vi "test1-HexStr conversion.vi"(8 "error in (no error)":errorcluster, 11 "TestCase in":refnum<class "testcase-CSMArgument.lvclass">) -> (0 "error out":errorcluster, 3 "TestCase out":refnum<class "testcase-CSMArgument.lvclass">)   [LabVIEW 2017, in "testcase-CSMArgument.lvclass"]
uses:
  testcase-CSMArgument.lvclass
  <vilib>/addons/_JKI Toolkits/VI Tester/TestCase.llb/TestCase.lvclass
  src/user.lib/_NEVSTOP/Communicable State Machine(CSM)/Communicable State Machine.lvlib
  src/user.lib/_NEVSTOP/Communicable State Machine(CSM)/_Shared/CSM Shared.lvlib
  CSM/CSM-Testcase.lvlib
  C:/Program Files (x86)/National Instruments/LabVIEW 2017/vi.lib/addons/_JKI Toolkits/VI Tester/TestCase.llb/TestCase.lvclass
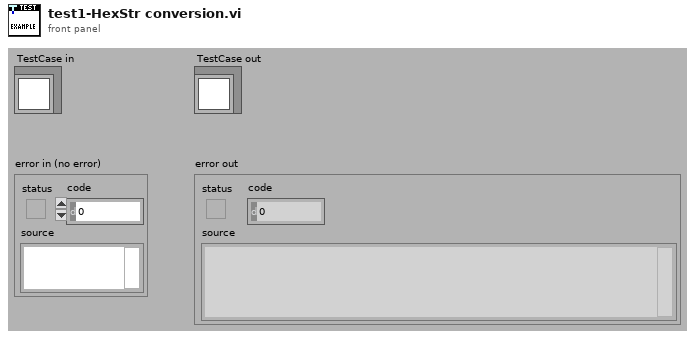
[diagram p1: front panel]
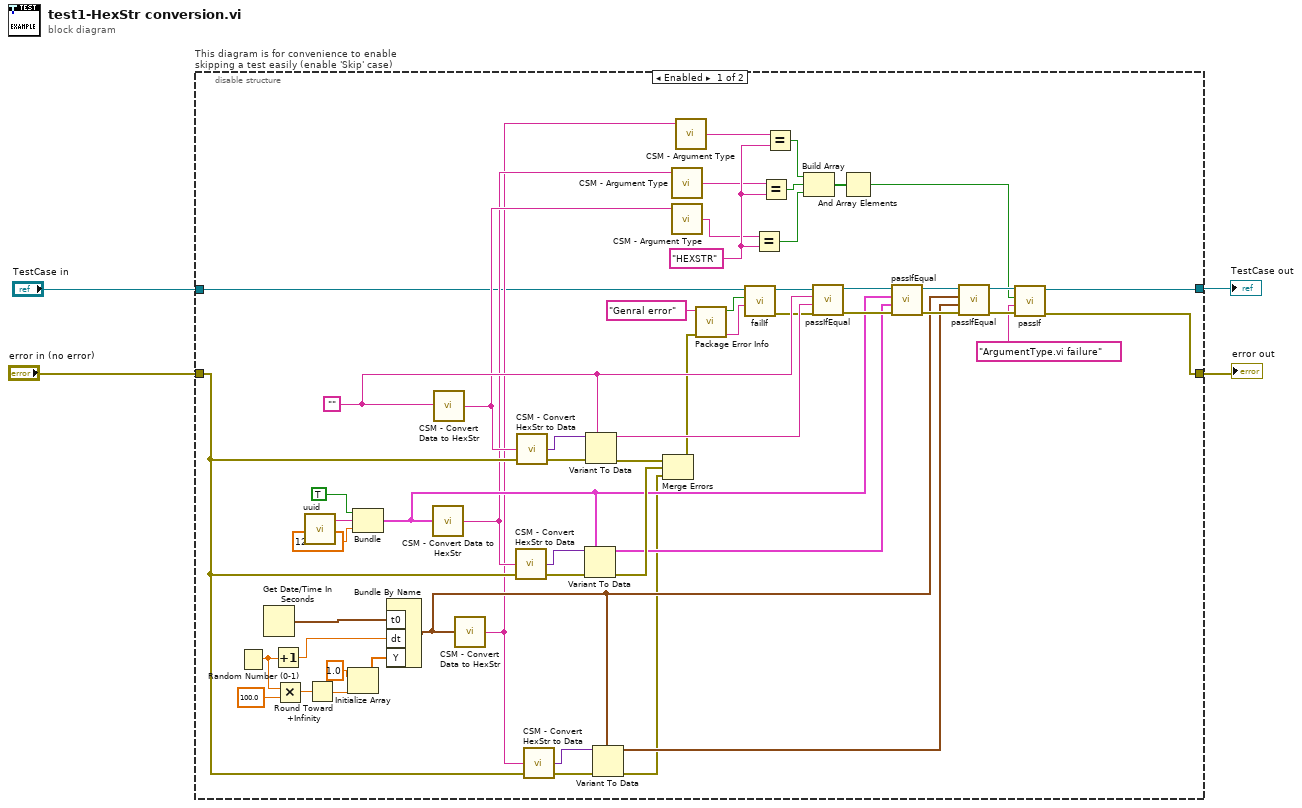
[diagram p0: block diagram]
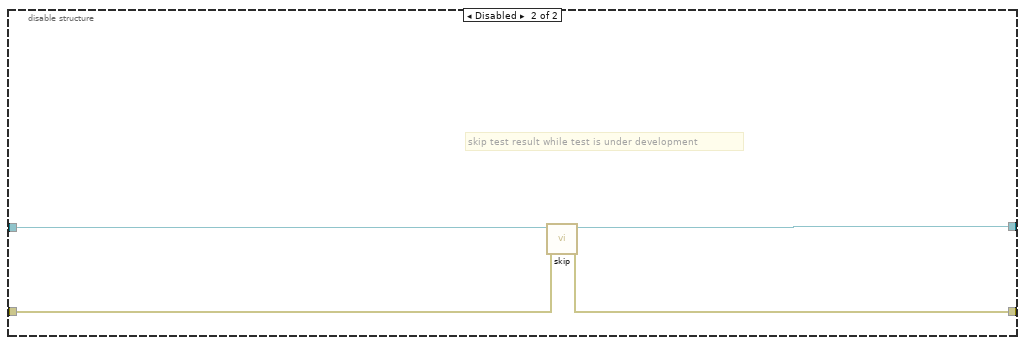
[diagram p2: hidden frame]
diagram:
  n1 = disable-structure "This diagram is for convenience to enable skipping a test easily (enable 'Skip' case)" shown="Enabled" {
    disable-tunnel: "TestCase in" -> [w11 w63]
    disable-tunnel: [w19 w61] -> w1
    disable-tunnel: [w17 w62] -> w3
    disable-tunnel: "error in (no error)" -> [w42 w60]
    frame Enabled {
      w25 = "HEXSTR"
      w53 = ""
      n2 = Random Number (0-1)() -> (number: 0 to 1=w38:dbl)
      n3 = Get Date/Time In Seconds() -> (seconds since 1Jan1904=w41:timestamp)
      n4 = Increment(x=w38) -> (x+1=w40:dbl)
      n5 = Multiply(x=w38, y=100.0) -> (x*y=w36:dbl)
      n6 = call "uuid.vi"() -> ("UUID"=w58:string)  [unwired: 11 in]
      n7 = Round Toward +Infinity(x=w36) -> (ceil(x): smallest int >= x=w35:dbl)
      n8 = Initialize Array(1.0 ("element"), w35) -> (w34:dbl[])
      n9 = Bundle(TRUE, "UUID"=w58, 123.456) -> (w46:cluster{bool, "UUID":string, dbl})  [unwired: 1 in]
      n10 = Bundle By Name("t0"=w41, "dt"=w40, "Y"=w34) -> (w31:waveform(dbl))  [unwired: 1 in]
      n11 = call "CSM - Convert Data to HexStr.vi"("Variant"=w46) -> ("HEX String (0-9,A-F)"=w27:string)  [unwired: 8 in]
      n12 = call "CSM - Convert Data to HexStr.vi"("Variant"=w53) -> ("HEX String (0-9,A-F)"=w28:string)  [unwired: 8 in]
      n13 = call "CSM - Convert Data to HexStr.vi"("Variant"=w31) -> ("HEX String (0-9,A-F)"=w26:string)  [unwired: 8 in]
      n14 = call "CSM - Convert HexStr to Data.vi"("HEX String"=w27, "error in (no error)"=w42) -> ("Variant"=w49:variant, "error out"=w51:errorcluster)  [unwired: 6 in]
      n15 = call "CSM - Convert HexStr to Data.vi"("HEX String"=w28, "error in (no error)"=w42) -> ("Variant"=w54:variant, "error out"=w56:errorcluster)  [unwired: 6 in]
      n16 = call "CSM - Convert HexStr to Data.vi"("HEX String"=w26, "error in (no error)"=w42) -> ("Variant"=w44:variant, "error out"=w43:errorcluster)  [unwired: 6 in]
      n17 = Variant To Data(error in=w51, type=w46, Variant=w49) -> (data=w45:cluster{bool, "UUID":string, dbl}, error out=w50:errorcluster)
      n18 = Variant To Data(error in=w56, type=w53, Variant=w54) -> (data=w52:string, error out=w55:errorcluster)
      n19 = Variant To Data(error in=w43, type=w31, Variant=w44) -> (data=w30:waveform(dbl), error out=w29:errorcluster)
      n20 = Merge Errors(w55, w50, w29) -> (w5:errorcluster)
      n21 = call "CSM - Argument Type.vi"("Arguments"=w27) -> ("Argument Type"=w15:string)  [unwired: 3 in, 1 out]
      n22 = call "CSM - Argument Type.vi"("Arguments"=w28) -> ("Argument Type"=w14:string)  [unwired: 3 in, 1 out]
      n23 = call "CSM - Argument Type.vi"("Arguments"=w26) -> ("Argument Type"=w12:string)  [unwired: 3 in, 1 out]
      n24 = call "Package Error Info.vi"("error in"=w5, "String in"="Genral error") -> ("packed error info out"=w7:string, "error status"=w8:bool)  [unwired: 8 in]
      n25 = call-dynamic "failIf.vi"("message (\"\")"=w7, "fail"=w8, "TestCase in"=w11) -> ("error out"=w9:errorcluster, "TestCase out"=w10:refnum<class "testcase-CSMArgument.lvclass">)  [unwired: 7 in]
      n26 = Equal?(x=w14, y=w25) -> (x = y?=w22:bool)
      n27 = Equal?(x=w15, y=w25) -> (x = y?=w24:bool)
      n28 = Equal?(x=w12, y=w25) -> (x = y?=w23:bool)
      n29 = Build Array(w23, w24, w22) -> (w21:bool[])
      n30 = call-dynamic "passIfEqual.vi"("error in (no error)"=w9, "y"=w52, "x"=w53, "TestCase in"=w10) -> ("error out"=w47:errorcluster, "TestCase out"=w48:refnum<class "testcase-CSMArgument.lvclass">)  [unwired: 6 in]
      n31 = And Array Elements(Boolean array=w21) -> (logical AND=w16:bool)
      n32 = call-dynamic "passIfEqual.vi"("error in (no error)"=w47, "y"=w45, "x"=w46, "TestCase in"=w48) -> ("error out"=w32:errorcluster, "TestCase out"=w33:refnum<class "testcase-CSMArgument.lvclass">)  [unwired: 6 in]
      n33 = call-dynamic "passIfEqual.vi"("error in (no error)"=w32, "y"=w30, "x"=w31, "TestCase in"=w33) -> ("error out"=w18:errorcluster, "TestCase out"=w20:refnum<class "testcase-CSMArgument.lvclass">)  [unwired: 6 in]
      n34 = call-dynamic "passIf.vi"("error in (no error)"=w18, "message (\"\")"="ArgumentType.vi failure", "pass"=w16, "TestCase in"=w20) -> ("error out"=w17:errorcluster, "TestCase out"=w19:refnum<class "testcase-CSMArgument.lvclass">)  [unwired: 6 in]
    }
    frame Disabled {
      # "skip test result while test is under development"
      n35 = call <vilib>:"skip.vi"("error in (no error)"=w60, "TestCase in"=w63) -> ("error out"=w62:errorcluster, "TestCase out"=w61:refnum<class "testcase-CSMArgument.lvclass">)  [unwired: 8 in]
    }
  }
  "error out" <- w3
  "TestCase out" <- w1
